vi "Http.vi"() -> ()   [LabVIEW 2023]
uses:
  <vilib>/httpClient/LabVIEWHTTPClient.lvlib
panel:
  out "Waveform Graph":dbl[](graph)
  out "body":string
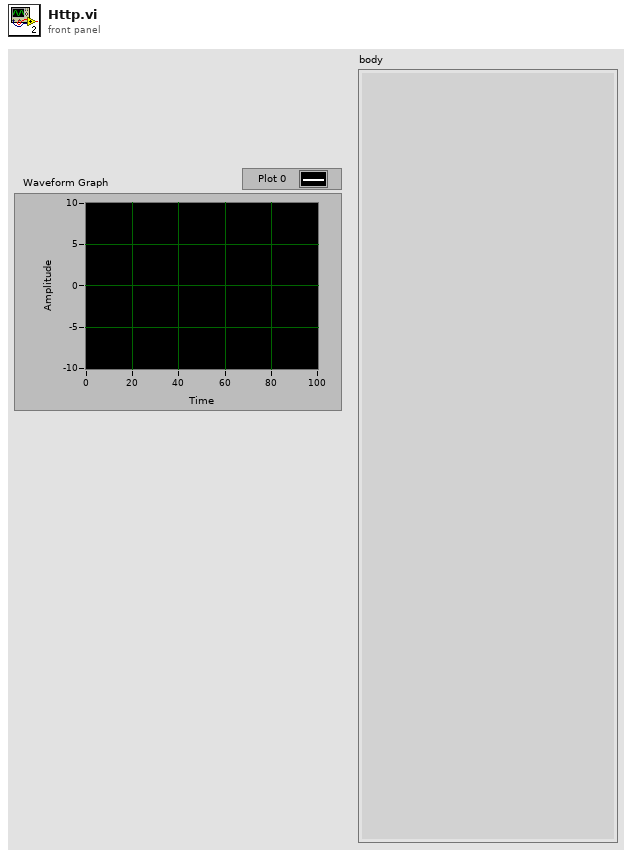
[diagram p1: front panel]
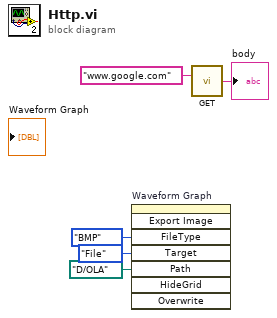
[diagram p0: block diagram]
diagram:
  n1 = invoke on="Waveform Graph" class="WFGraph (strict)" method="Export Image"("FileType"=enum32{"BMP", "EPS", "EMF", "PICT"}."BMP" ("File Type"), "Target"=enum32{"File", "Clipboard"}."File", "Path"=path "D:/OLA") -> ()  [unwired: 5 in, 8 out]
  n2 = call <vilib>:"GET.vi"("url"="www.google.com") -> ("body"=→"body":string)  [unwired: 11 in, 3 out]
